vi "Reply Msg DataSocket Simple.vi"(8 "error in (no error)":errorcluster, 10 "Input":variant, 11 "Target Reply Time Test Actor in":refnum<class "Target Reply Time Test Actor.lvclass">) -> (0 "error out":errorcluster, 2 "Reply":variant, 3 "Target Reply Time Test Actor out":refnum<class "Target Reply Time Test Actor.lvclass">)   [LabVIEW 2023, in "Target Reply Time Test Actor.lvlib" / "Target Reply Time Test Actor.lvclass"]
uses:
  Target Reply Time Test Actor.lvclass
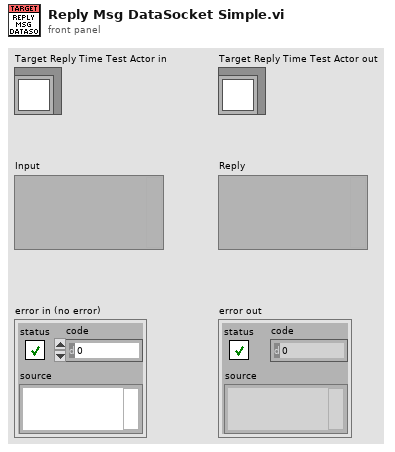
[diagram p1: front panel]
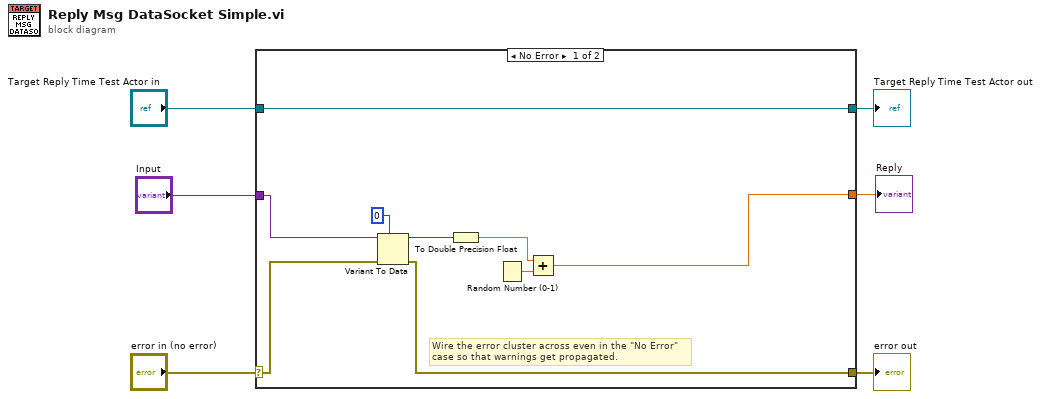
[diagram p0: block diagram]
diagram:
  n1 = case shown="No Error" "error in (no error)" {
    selector: "error in (no error)" -> [w13 w17]
    tunnel: [w12 w17] -> w5
    tunnel: [w15 w16] -> w3
    tunnel: "Target Reply Time Test Actor in" -> [w15 w16]
    tunnel: [w7 _] -> w2
    tunnel: "Input" -> [w10 _]
    frame No Error {
      # "Wire the error cluster across even in the \"No Error\"\ncase so that warnings get propagated."
      n2 = Variant To Data(error in=w13, type=0, Variant=w10) -> (data=w9:i32, error out=w12:errorcluster)
      n3 = To Double Precision Float(number=w9) -> (double precision float=w8:dbl)
      n4 = Random Number (0-1)() -> (number: 0 to 1=w14:dbl)
      n5 = Add(x=w8, y=w14) -> (x+y=w7:dbl)
    }
    frame Error {
    }
  }
  "error out" <- w5
  "Target Reply Time Test Actor out" <- w3
  "Reply" <- w2
